vi "Write Class Data.vi"(6 "Remote Address":string, 8 "error in (no error)":errorcluster, 9 "Message Broker":refnum<class "Message Broker Interface.lvclass">, 10 "Connection ID":refnum<k5>, 11 "Websocket Client Handler in":refnum<class "Websocket Client Handler.lvclass">) -> (0 "error out":errorcluster, 3 "Websocket Client Handler out":refnum<class "Websocket Client Handler.lvclass">)   [LabVIEW 2016, in "Stream Mediator.lvlib" / "Websocket Client Handler.lvclass"]
doc: "--\nCopyright © 2017 Composed SystemsI All rights reserved.\n\nAuthor: Jon McBee <jon.mcbee@composed.io>\n\nThis library is provided \"AS IS\" ,WITHOUT WARRANTIES OR\nCONDITIONS OF ANY KIND, either express or implied.\n\nComposed Systems -- composed.io\n\nStream 0.0.1.1\nJon McBee - Composed Systems\nCopyright (c) 2017, Composed Systems"
uses:
  <userlib>/Composed Systems/Stream/Mediator/Classes/Websocket Client Handler Actor/Websocket Client Handler/Websocket Client Handler.lvclass
  C:/Program Files (x86)/National Instruments/LabVIEW 2016/user.lib/Composed Systems/Stream/Mediator/Classes/Mediated Actor/Mediated Actor.lvclass
  <userlib>/Composed Systems/Stream/Mediator/Classes/Message Broker Interface/Message Broker Interface.lvclass
  <userlib>/Composed Systems/Stream/Mediator/Classes/Websocket Client Handler Actor/Websocket Client Handler/Websocket Client Handler.lvclass/Websocket Client Handler.ctl
  <userlib>/Composed Systems/Stream/Mediator/Classes/Mediated Actor/Mediated Actor.lvclass
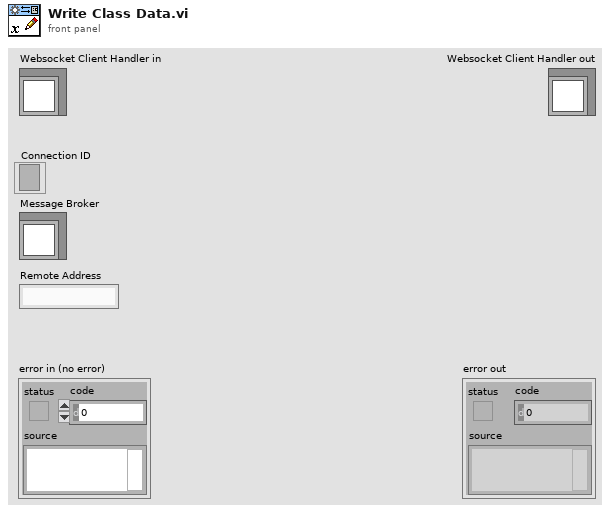
[diagram p1: front panel]
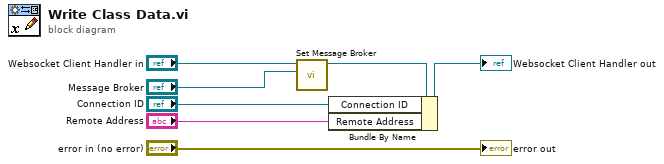
[diagram p0: block diagram]
diagram:
  n1 = call <userlib>:"Set Message Broker.vi"("Message Broker"="Message Broker", "Mediated Actor in"="Websocket Client Handler in") -> ("Mediated Actor out"=w2:refnum<class "Websocket Client Handler.lvclass">)  [unwired: 9 in]
  n2 = Bundle By Name(cluster=w2, "Connection ID"="Connection ID", "Remote Address"="Remote Address") -> (→"Websocket Client Handler out":refnum<class "Websocket Client Handler.lvclass">)
  "error out" <- "error in (no error)"
